vi "MULTTCP2_AsyncHandler.vi"(0 "async_on_block":refnum<vi>, 1 "last async ref":refnum<vi>, 5 "block notifier":refnum<notifier>, 7 "asyncN":refnum<notifier>, 9 "async notifier":refnum<notifier>, 11 "error async out":errorcluster, 12 "async reference":refnum<vi>, 13 "logfile":path, 14 "Log":bool=TRUE) -> (15 "error async out":errorcluster)   [LabVIEW 2016]
uses:
  DBSHAND/private/vis/DatabaseHand_Element_Get(string).vi
panel:
  in  "async_on_block 2":bool
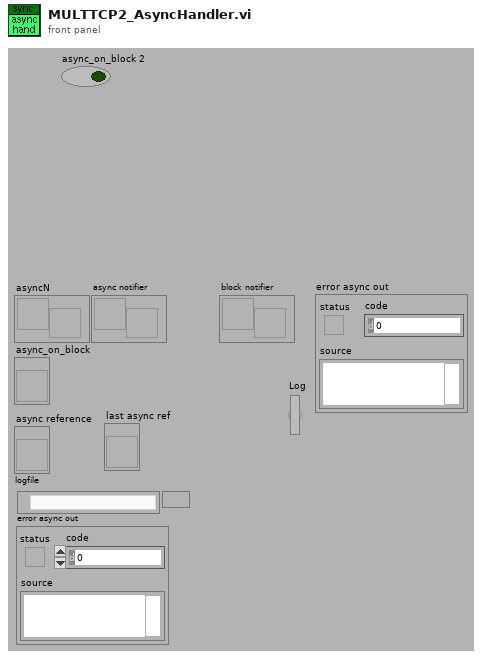
[diagram p1: front panel]
types:
  T1 = typedef "DatabaseHand_RefNum.ctl" = refnum<vi>
  T2 = typedef "MULTTCP2_BlockingStruct.ctl" = cluster{"cmd":string, "message back  queue":refnum<queue>}
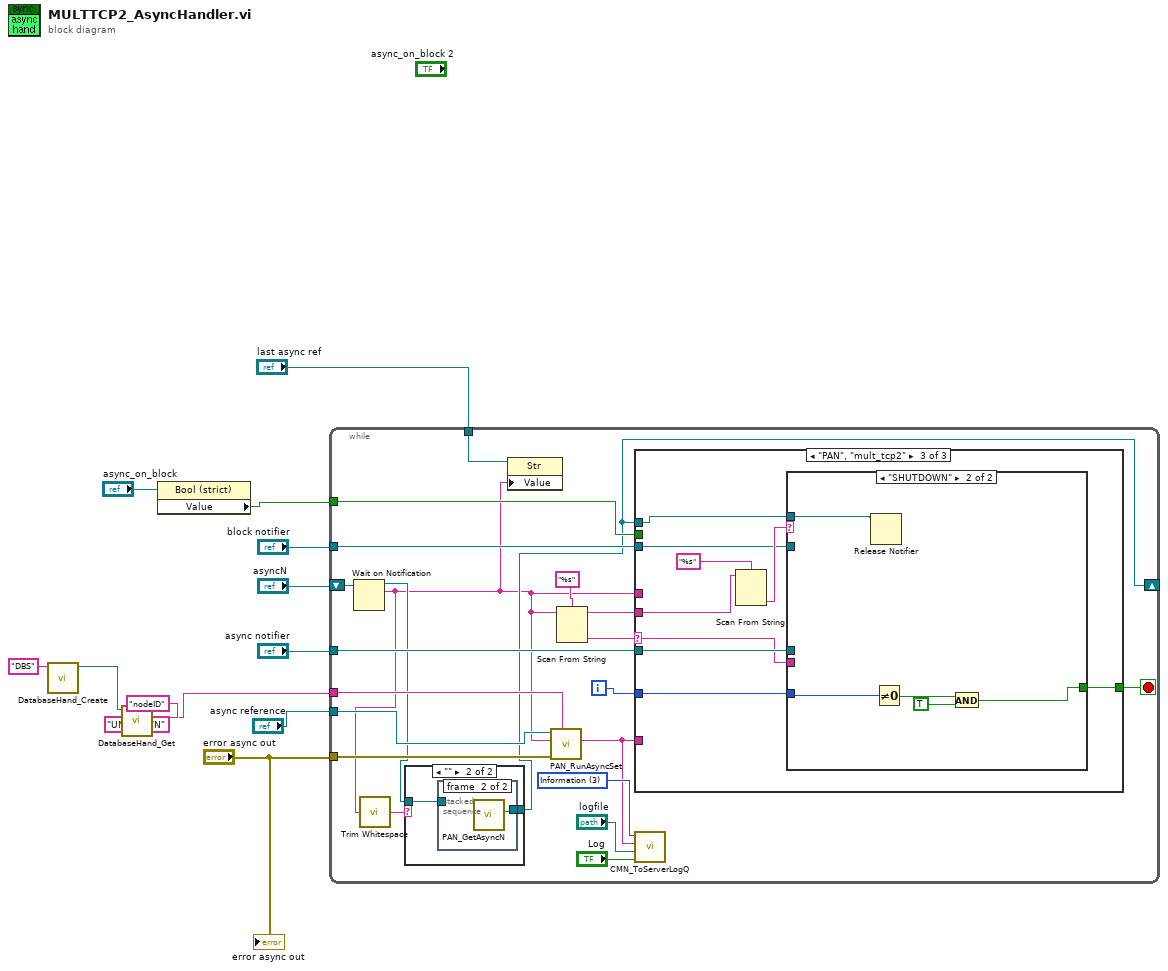
[diagram p0: block diagram]
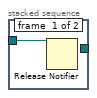
[diagram p3: hidden frame]
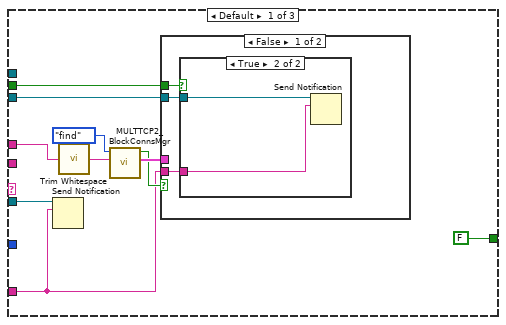
[diagram p4: hidden frame]
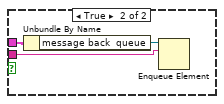
[diagram p6: hidden frame]
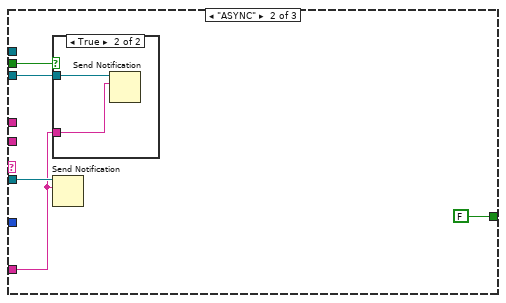
[diagram p7: hidden frame]
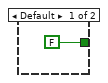
[diagram p9: hidden frame]
diagram:
  n1 = call "DatabaseHand_Create.vi"("Name"="DBS") -> ("Database RefNum out"=w3:T1)  [unwired: 1 in, 9 out]
  n2 = call-poly "DatabaseHand_Get.vi"("default value"="UNKNOWN", "name"="nodeID", "Database RefNum in"=w3) -> ("value"=w2:string)  [unwired: 2 in, 6 out]
  n3 = property class="Bool (strict)"(reference="async_on_block") -> ("Value"=w6:bool)  [unwired: 1 in, 2 out]
  n4 = while {
    tunnel: "async notifier" -> [w31]
    tunnel: "block notifier" -> [w28]
    tunnel: "async reference" -> [w27]
    tunnel: "error async out" -> [w26]
    tunnel: w6 -> [w24]
    tunnel: "last async ref" -> [w21]
    tunnel: w2 -> [w20]
    shift-right: [w16] -> _
    shift-left: "asyncN" -> [w18]
    i -> [w19]
    stop <- w32 stop-if-true
    w29 = u16 3 items=["command", "imediateReply", "Callback Reply", "Information", "none"] ("type")
    n5 = Wait on Notification(notifier=w18) -> (notifier out=w17:refnum<notifier>, notification=w14:string)  [unwired: 1 in, 4 out]
    n6 = call <vilib>:"Trim Whitespace.vi"("string"=w14) -> ("trimmed string"=w15:string)  [unwired: 1 in]
    n7 = case shown="\"\"" w15 {
      tunnel: w17 -> [w35 w37]
      tunnel: [w35 w36] -> w16
      frame Default {
      }
      frame "" {
        n8 = stacked-sequence {
          tunnel: w37 -> [w38 _]
          tunnel: [_ w39] -> w36
          frame #0 {
            n9 = Release Notifier(notifier=w38) -> ()  [unwired: 1 in, 4 out]
          }
          frame #1 {
            n10 = call "PAN_GetAsyncN.vi"() -> ("asyncN"=w39:refnum<notifier>)  [unwired: 11 out]
          }
        }
      }
    }
    n11 = property class="Str"(reference=w21, "Value"=w14) -> ()  [unwired: 1 in, 2 out]
    n12 = call "PAN_RunAsyncSet.vi"("nodeID"=w20, "error in (no error)"=w26, "msg in"=w14, "type specifier VI Refnum (for type only)"=w27) -> ("resp out"=w25:string)  [unwired: 7 out]
    n13 = Scan From String(format string="%s", input string=w14) -> (remaining string=w30:string, output 1=w33:string)  [unwired: 2 in, 3 out]
    n14 = case shown="\"PAN\", \"mult_tcp2\"" w33 {
      selector: w33 -> [_ _ w72]
      tunnel: [FALSE FALSE w68] -> w32
      tunnel: w31 -> [w42 w61 w73]
      tunnel: w14 -> [w46 _ _]
      tunnel: w16 -> [_ _ w66]
      tunnel: w30 -> [_ _ w71]
      tunnel: w28 -> [w41 w60 w67]
      tunnel: w25 -> [w43 w59 _]
      tunnel: w24 -> [w40 w58 _]
      tunnel: w19 -> [_ _ w65]
      frame Default {
        n15 = Send Notification(notification=w43, notifier=w42) -> ()  [unwired: 1 in, 2 out]
        n16 = call <vilib>:"Trim Whitespace.vi"("string"=w46) -> ("trimmed string"=w45:string)  [unwired: 1 in]
        n17 = call "MULTTCP2_BlockConnsMgr.vi"("arg"=w45, "action"=enum16{"add", "delete", "find"}."find") -> ("connection out"=w48:T2, "send CB"=w44:bool)  [unwired: 2 in, 6 out]
        n18 = case shown="False" w44 {
          tunnel: w48 -> [_ w57]
          tunnel: w43 -> [w51 w55]
          tunnel: w41 -> [w52 _]
          tunnel: w40 -> [w50 _]
          frame False {
            n19 = case shown="True" w50 {
              tunnel: w52 -> [_ w54]
              tunnel: w51 -> [_ w53]
              frame False {
              }
              frame True {
                n20 = Send Notification(notification=w53, notifier=w54) -> ()  [unwired: 1 in, 2 out]
              }
            }
          }
          frame True {
            n21 = Unbundle By Name(w57) -> ("message back  queue"=w56:refnum<queue>)
            n22 = Enqueue Element(queue=w56, element=w55) -> ()  [unwired: 1 in, 4 out]
          }
        }
      }
      frame "ASYNC" {
        n23 = case shown="True" w58 {
          tunnel: w60 -> [_ w64]
          tunnel: w59 -> [_ w63]
          frame False {
          }
          frame True {
            n24 = Send Notification(notification=w63, notifier=w64) -> ()  [unwired: 1 in, 2 out]
          }
        }
        n25 = Send Notification(notification=w59, notifier=w61) -> ()  [unwired: 1 in, 2 out]
      }
      frame "PAN", "mult_tcp2" {
        n26 = Scan From String(format string="%s", input string=w71) -> (output 1=w69:string)  [unwired: 2 in, 4 out]
        n27 = case shown="\"SHUTDOWN\"" w69 {
          tunnel: w73 -> [_ _]
          tunnel: w72 -> [_ _]
          tunnel: [FALSE w75] -> w68
          tunnel: w67 -> [_ _]
          tunnel: w66 -> [_ w79]
          tunnel: w65 -> [_ w78]
          frame Default {
          }
          frame "SHUTDOWN" {
            n28 = Release Notifier(notifier=w79) -> ()  [unwired: 1 in, 4 out]
            n29 = Not Equal To 0?(x=w78) -> (x != 0?=w77:bool)
            n30 = And(x=w77, y=TRUE) -> (x .and. y?=w75:bool)
          }
        }
      }
    }
    n31 = call "CMN_ToServerLogQ.vi"("Log"="Log", "file"="logfile", "string"=w25, "type"=w29) -> ()  [unwired: 2 in, 5 out]
  }
  "error async out" <- "error async out"
